vi "Enter Field.vi"(7 "Field monitor":refnum<vi>, 8 "error in (no error)":errorcluster, 9 "Abort button":refnum<vi>, 10 "Target field":dbl[unit], 11 "Power Supply in":refnum<class "Power Supply.lvclass">) -> (0 "error out":errorcluster, 3 "Power Supply out":refnum<class "Power Supply.lvclass">)   [LabVIEW 2009, in "Power Supply.lvclass"]
doc: "Establish an initial magnetic field - perhaps starting at zero or some other point. Use this SubVI for large (not incremental) field adjustments."
uses:
  Power Supply.lvclass
  Power Supply.lvclass/Power Supply.ctl
  Global/Sound Files.vi
panel:
  in  "Dummy field monitor":dbl[unit]
  in  "Status display":refnum<vi>
  in  "resetrate?":bool
  out "canceled?":bool
  in  "cancel":bool
  out "disp":string
  out "fieldOUT":dbl[unit]
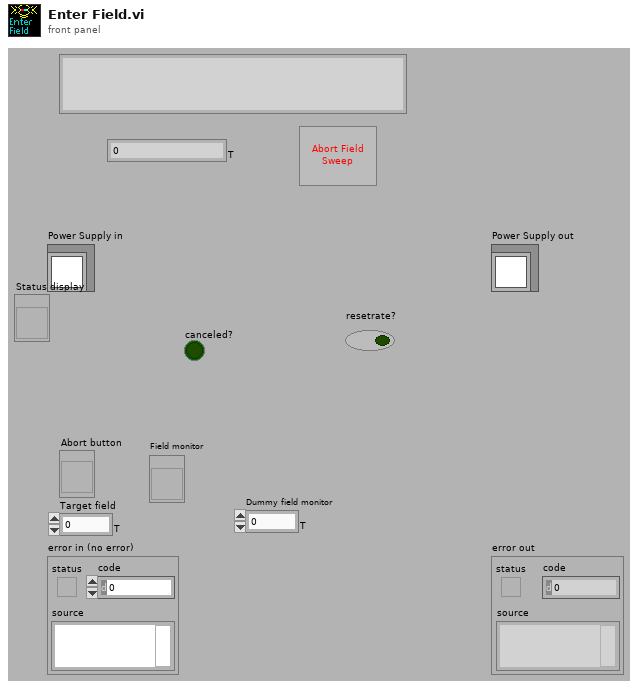
[diagram p1: front panel]
types:
  T1 = typedef "Power Supply.lvclass/Ramping Mode.ctl" = enum16{"Train Speed", "Maximum Speed", "Manual"}
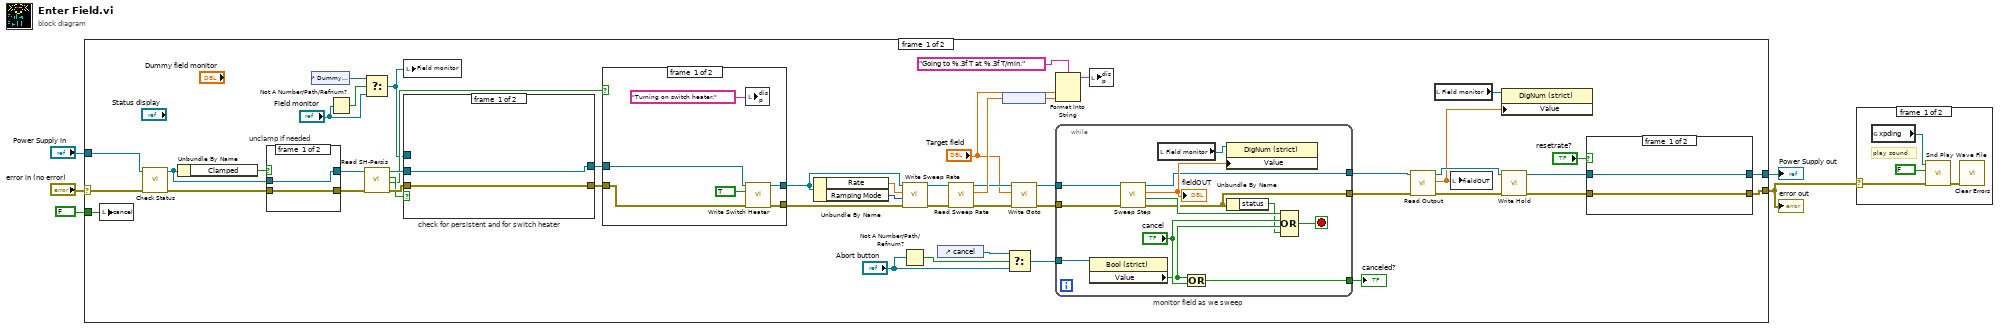
[diagram p0: block diagram]
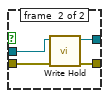
[diagram p4: hidden frame]
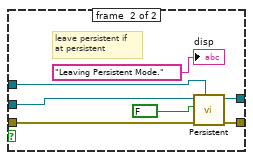
[diagram p5: hidden frame]
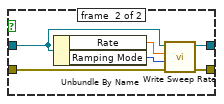
[diagram p6: hidden frame]
diagram:
  n1 = case shown="No Error" "error in (no error)" {
    selector: "error in (no error)" -> [w13 w100]
    tunnel: [w54 w100] -> w1
    tunnel: [w53 w99] -> w5
    tunnel: "Power Supply in" -> [w52 w99]
    tunnel: FALSE ("cancel") -> [w11 _]
    frame #0 {
      n2 = local write "cancel"(w11) -> ()
      n3 = call-dynamic "Check Status.vi"("error in (no error)"=w13, "Power Supply in"=w52) -> ("error out"=w21:errorcluster, "Power Supply out"=w22:refnum<class "Power Supply.lvclass">)  [unwired: 6 in, 2 out]
      n4 = Unbundle By Name(w22) -> ("Clamped"=w23:bool)
      n5 = case "unclamp if needed" shown="False" w23 {
        tunnel: w22 -> [w64 w68]
        tunnel: [w64 w67] -> w28
        tunnel: w21 -> [w63 w66]
        tunnel: [w63 w65] -> w27
        frame #0 {
        }
        frame #1 {
          n6 = call-dynamic "Write Hold.vi"("error in (no error)"=w66, "Power Supply in"=w68) -> ("error out"=w65:errorcluster, "Power Supply out"=w67:refnum<class "Power Supply.lvclass">)  [unwired: 8 in]
        }
      }
      n7 = control-ref of="Dummy field monitor"() -> (w7:refnum<vi>)
      n8 = Not A Number/Path/Refnum?(number/path/refnum="Field monitor") -> (NaN/Path/Refnum?=w9:bool)
      n9 = Select(t=w7, s=w9, f="Field monitor") -> (s? t:f=w6:refnum<vi>)
      n10 = call-dynamic "Read SH-Persis.vi"("error in (no error)"=w27, "Power Supply in"=w28) -> ("error out"=w25:errorcluster, "SHon?"=w14:bool, "pers?"=w24:bool, "Power Supply out"=w26:refnum<class "Power Supply.lvclass">)  [unwired: 4 in, 2 out]
      n11 = local write "Field monitor"(w6) -> ()
      n12 = case "check for persistent and for switch heater" shown="False" w24 {
        tunnel: w26 -> [w70 w73]
        tunnel: [w70 w74] -> w18
        tunnel: w25 -> [w69 w76]
        tunnel: [w69 w75] -> w17
        tunnel: w6 -> [_ w71]
        frame #0 {
        }
        frame #1 {
          # "leave persistent if\nat persistent"
          n13 = call-dynamic "Persistent.vi"("Field monitor ref"=w71, "error in (no error)"=w76, "Go to persistent mode?"=FALSE, "Power Supply in"=w73) -> ("error out"=w75:errorcluster, "Power Supply out"=w74:refnum<class "Power Supply.lvclass">)  [unwired: 6 in]
          "disp" <- "Leaving Persistent Mode."
        }
      }
      n14 = case shown="True" w14 {
        tunnel: w18 -> [w60 w61]
        tunnel: [w59 w61] -> w16
        tunnel: w17 -> [w58 w62]
        tunnel: [w57 w62] -> w15
        frame #0 {
          n15 = local write "disp"("Turning on switch heater." ("disp")) -> ()
          n16 = call-dynamic "Write Switch Heater.vi"("error in (no error)"=w58, "Turn SH On?"=TRUE, "Power Supply in"=w60) -> ("error out"=w57:errorcluster, "Power Supply out"=w59:refnum<class "Power Supply.lvclass">)  [unwired: 7 in]
        }
        frame #1 {
        }
      }
      n17 = Unbundle By Name(w16) -> ("Rate"=w20:dbl[unit], "Ramping Mode"=w19:T1)
      n18 = Not A Number/Path/Refnum?(number/path/refnum="Abort button") -> (NaN/Path/Refnum?=w40:bool)
      n19 = call-dynamic "Write Sweep Rate.vi"("error in (no error)"=w15, "Ramping Mode"=w19, "rate"=w20, "Power Supply in"=w16) -> ("error out"=w31:errorcluster, "Power Supply out"=w32:refnum<class "Power Supply.lvclass">)  [unwired: 6 in]
      n20 = control-ref of="cancel"() -> (w37:refnum<vi>)
      n21 = call-dynamic "Read Sweep Rate.vi"("error in (no error)"=w31, "Power Supply in"=w32) -> ("error out"=w29:errorcluster, "Field sweep rate"=w49:dbl[unit], "Power Supply out"=w30:refnum<class "Power Supply.lvclass">)  [unwired: 7 in]
      n22 = node(w49) -> (w12:dbl)
      n23 = Select(t=w37, s=w40, f="Abort button") -> (s? t:f=w38:refnum<vi>)
      n24 = call-dynamic "Write Goto.vi"("error in (no error)"=w29, "Target"="Target field", "Power Supply in"=w30) -> ("error out"=w36:errorcluster, "Power Supply out"=w35:refnum<class "Power Supply.lvclass">)  [unwired: 7 in]
      n25 = Format Into String(format string="Going to %.3f T at %.3f T/min.", "Target field", w12) -> (resulting string=w33:string)  [unwired: 2 in, 1 out]
      n26 = while "monitor field as we sweep" {
        tunnel: w38 -> [w87]
        tunnel: w36 -> [w86]
        tunnel: w35 -> [w85]
        tunnel: [w79] -> w44
        tunnel: [w84] -> w43
        tunnel: [w81] -> w45
        stop <- w90 stop-if-true
        n27 = property on="Property Node" class="Bool (strict)"(reference=w87) -> ("Value"=w82:bool)  [unwired: 1 in, 2 out]
        n28 = call-dynamic "Sweep Step.vi"("error in (no error)"=w86, "Power Supply in"=w85) -> ("error out"=w79:errorcluster, "Done?"=w89:bool, "field"=w88:dbl[unit], "Power Supply out"=w84:refnum<class "Power Supply.lvclass">)  [unwired: 6 in]
        "fieldOUT" <- w88
        n29 = local read "Field monitor"() -> (w80:refnum<vi>)
        n30 = Compound Arithmetic op=OR(w82, "cancel") -> (w81:bool)
        n31 = property class="DigNum (strict)"(reference=w80, "Value"=w88) -> ()  [unwired: 1 in, 2 out]
        n32 = Unbundle By Name(w79) -> ("status"=w78:bool)
        n33 = Compound Arithmetic op=OR(w89, "cancel", w82, w78) -> (w90:bool)
      }
      "canceled?" <- w45
      n34 = local write "disp"(w33) -> ()
      n35 = call-dynamic "Read Output.vi"("error in (no error)"=w44, "Power Supply in"=w43) -> ("error out"=w46:errorcluster, "Field"=w41:dbl[unit], "Power Supply out"=w47:refnum<class "Power Supply.lvclass">)  [unwired: 6 in, 1 out]
      n36 = local read "Field monitor"() -> (w42:refnum<vi>)
      n37 = local write "fieldOUT"(w41) -> ()
      n38 = property class="DigNum (strict)"(reference=w42, "Value"=w41) -> ()  [unwired: 1 in, 2 out]
      n39 = call-dynamic "Write Hold.vi"("error in (no error)"=w46, "Power Supply in"=w47) -> ("error out"=w48:errorcluster, "Power Supply out"=w50:refnum<class "Power Supply.lvclass">)  [unwired: 8 in]
      n40 = case shown="True" "resetrate?" {
        tunnel: w50 -> [w92 w95]
        tunnel: w48 -> [w91 w98]
        tunnel: [w91 w97] -> w54
        tunnel: [w92 w96] -> w53
        frame #0 {
        }
        frame #1 {
          n41 = Unbundle By Name(w95) -> ("Rate"=w94:dbl[unit], "Ramping Mode"=w93:T1)
          n42 = call-dynamic "Write Sweep Rate.vi"("error in (no error)"=w98, "Ramping Mode"=w93, "rate"=w94, "Power Supply in"=w95) -> ("error out"=w97:errorcluster, "Power Supply out"=w96:refnum<class "Power Supply.lvclass">)  [unwired: 6 in]
        }
      }
    }
    frame #1 {
    }
  }
  "error out" <- w1
  "Power Supply out" <- w5
  n43 = case shown="No Error" w1 {
    selector: w1 -> [w102 _]
    frame #0 {
      # "play sound"
      n44 = global read "Sound Files.vi" "xpding"() -> (w103:path)
      n45 = call <vilib>:"Snd Play Wave File.vi"("error in (no error)"=w102, "wait until finish (T)"=FALSE, "wave file path"=w103) -> ("error out"=w101:errorcluster)  [unwired: 8 out]
      n46 = call <vilib>:"Clear Errors.vi"("error in (no error)"=w101) -> ()  [unwired: 6 in, 1 out]
    }
    frame #1 {
    }
  }
